vi "FRANCELINO_VI01.vi"(9 "Nota VC":dbl, 11 "Notas de VE":dbl[](array[numeric])) -> (3 "Nota de VF":dbl)   [LabVIEW 2018]
panel:
  out "Media de VE":dbl
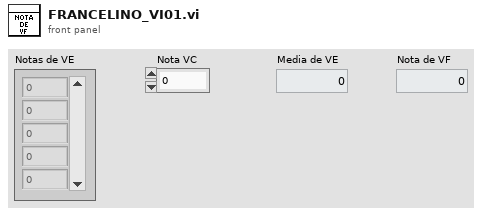
[diagram p1: front panel]
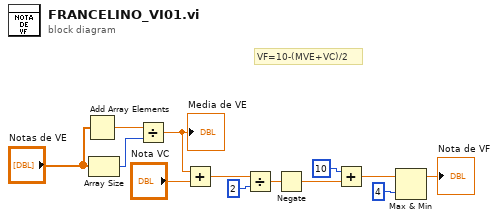
[diagram p0: block diagram]
diagram:
  # "VF=10-(MVE+VC)/2"
  n1 = Add Array Elements(numeric array="Notas de VE") -> (sum=w12:dbl)
  n2 = Array Size(array="Notas de VE") -> (size(s)=w11:i32)
  n3 = Divide(x=w12, y=w11) -> (x/y=w10:dbl)
  "Media de VE" <- w10
  n4 = Add(x=w10, y="Nota VC") -> (x+y=w9:dbl)
  n5 = Divide(x=w9, y=2) -> (x/y=w7:dbl)
  n6 = Negate(x=w7) -> (-x=w5:dbl)
  n7 = Add(x=10, y=w5) -> (x+y=w2:dbl)
  n8 = Max & Min(x=w2, y=4) -> (max(x,y)=→"Nota de VF":dbl)  [unwired: 1 out]
